vi "MandelbrotMain.vi"() -> ()   [LabVIEW 2013]
panel:
  out "milliseconds":dbl
  out "String":string
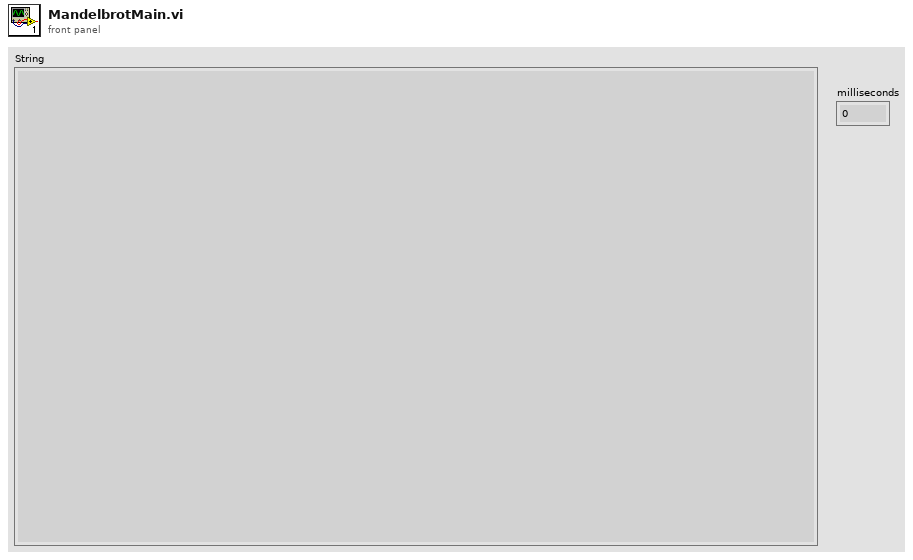
[diagram p1: front panel]
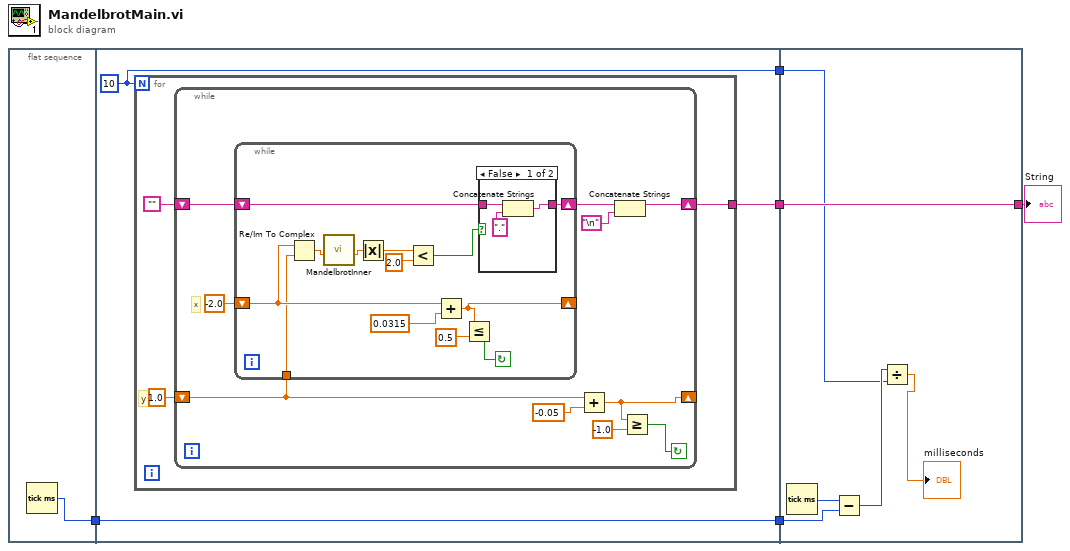
[diagram p0: block diagram]
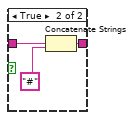
[diagram p2: hidden frame]
diagram:
  n1 = flat-sequence {
    tunnel: [w6] -> w5
    tunnel: w5 -> [w9]
    tunnel: [w9] -> w4
    tunnel: [w8] -> w2
    tunnel: [w7] -> w1
    tunnel: w4 -> [w46]
    tunnel: [w45] -> w3
    tunnel: w2 -> [w45]
    tunnel: w1 -> [w43]
    frame #0 {
      n2 = Tick Count (ms)() -> (millisecond timer value=w6:u32)
    }
    frame #1 {
      w7 = 10
      n3 = for {
        N: w7 -> [_]
        tunnel: [w10] -> w8
        # "y"
        n4 = while {
          shift-right: [w17] -> _
          shift-left: 1.0 -> [w14]
          shift-right: [w19] -> w10
          shift-left: "" -> [w20]
          stop <- w16 continue-if-true
          # "x"
          n5 = while {
            shift-right: [w34] -> _
            shift-left: -2.0 -> [w25]
            shift-right: [w30] -> w18
            shift-left: w20 -> [w31]
            tunnel: w14 -> [w24]
            stop <- w35 continue-if-true
            n6 = Re/Im To Complex(1:w24, 2:w25) -> (0:w29:cdb)
            n7 = call "MandelbrotInner.vi"("Numeric"=w29) -> ("Numeric 2"=w28:cdb)  [unwired: 6 in]
            n8 = Absolute Value(x=w28) -> (abs(x)=w27:dbl)
            n9 = Less?(x=w27, y=2.0) -> (x < y?=w23:bool)
            n10 = Add(x=w25, y=0.0315) -> (x+y=w34:dbl)
            n11 = Less Or Equal?(x=w34, y=0.5) -> (x <= y?=w35:bool)
            n12 = case shown="False" w23 {
              tunnel: w31 -> [w38 w41]
              tunnel: [w36 w40] -> w30
              frame False {
                n13 = Concatenate Strings(w38, ".") -> (w36:string)
              }
              frame True {
                n14 = Concatenate Strings(w41, "#") -> (w40:string)
              }
            }
          }
          n15 = Add(x=w14, y=-0.05) -> (x+y=w17:dbl)
          n16 = Concatenate Strings(w18, "\n") -> (w19:string)
          n17 = Greater Or Equal?(x=w17, y=-1.0) -> (x >= y?=w16:bool)
        }
      }
    }
    frame #2 {
      n18 = Tick Count (ms)() -> (millisecond timer value=w47:u32)
      n19 = Subtract(x=w47, y=w46) -> (x-y=w44:u32)
      n20 = Divide(x=w44, y=w43) -> (x/y=→"milliseconds":dbl)
    }
  }
  "String" <- w3
